vi "转换数组簇.vi"(0 "PLC采集值":T1) -> ()   [LabVIEW 2018]
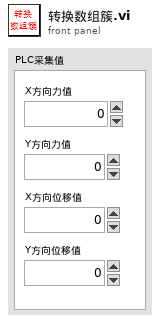
[diagram p1: front panel]
types:
  T1 = cluster{"X方向力值":sgl, "Y方向力值":sgl, "X方向位移值":sgl, "Y方向位移值":sgl}
  T2 = cluster{"Fx":sgl[], "Fy":sgl[], "Dx":sgl[], "Dy":sgl[]}
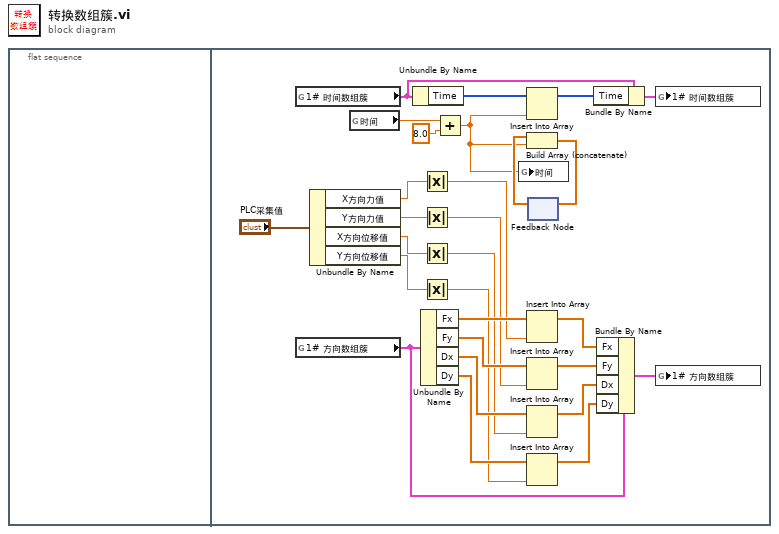
[diagram p0: block diagram]
diagram:
  n1 = flat-sequence {
    frame #0 {
    }
    frame #1 {
      n2 = global read "全局 1.vi" "1# 时间数组簇"() -> (w8:cluster{"Time":i32[]})
      n3 = global read "全局 1.vi" "1# 方向数组簇"() -> (w15:T2)
      n4 = Unbundle By Name("PLC采集值") -> ("X方向力值"=w27:sgl, "Y方向力值"=w23:sgl, "X方向位移值"=w22:sgl, "Y方向位移值"=w21:sgl)
      n5 = global read "全局 1.vi" "时间"() -> (w5:sgl)
      n6 = Unbundle By Name(w8) -> ("Time"=w9:i32[])
      n7 = Unbundle By Name(w15) -> ("Fx"=w14:sgl[], "Fy"=w26:sgl[], "Dx"=w25:sgl[], "Dy"=w24:sgl[])
      n8 = Absolute Value(x=w27) -> (abs(x)=w12:sgl)
      n9 = Absolute Value(x=w23) -> (abs(x)=w13:sgl)
      n10 = Absolute Value(x=w22) -> (abs(x)=w11:sgl)
      n11 = Absolute Value(x=w21) -> (abs(x)=w10:sgl)
      n12 = Add(x=w5, y=sgl 8.0) -> (x+y=w1:sgl)
      n13 = global write "全局 1.vi" "时间"(w1) -> ()
      n14 = Insert Into Array(array=w9, new element=w1) -> (w7:i32[])  [unwired: 1 in]
      n15 = Insert Into Array(array=w14, new element=w12) -> (w20:sgl[])  [unwired: 1 in]
      n16 = Insert Into Array(array=w26, new element=w13) -> (w19:sgl[])  [unwired: 1 in]
      n17 = Insert Into Array(array=w25, new element=w11) -> (w18:sgl[])  [unwired: 1 in]
      n18 = Insert Into Array(array=w24, new element=w10) -> (w17:sgl[])  [unwired: 1 in]
      n19 = feedback #1() -> (w2:sgl[])  [unwired: 1 in]
      n20 = Build Array (concatenate)(w2, w1) -> (w3:sgl[])
      n21 = feedback-in #1(w3) -> ()
      n22 = Bundle By Name(cluster=w8, "Time"=w7) -> (w6:cluster{"Time":i32[]})
      n23 = Bundle By Name(cluster=w15, "Fx"=w20, "Fy"=w19, "Dx"=w18, "Dy"=w17) -> (w16:T2)
      n24 = global write "全局 1.vi" "1# 时间数组簇"(w6) -> ()
      n25 = global write "全局 1.vi" "1# 方向数组簇"(w16) -> ()
    }
  }
